vi "subFindAndSetSourcePath.vi"(4 "Name":string, 6 "ProjectItem path":path, 7 "Owning project":path, 9 "Skip":bool, 11 "Project items in":T1) -> (1 "Found":bool, 2 "Item found":refnum<class "ProjectItem.lvclass">[](array[class]), 3 "Project items out":T1)   [LabVIEW 2020, in "SolutionBuilder.lvlib" / "SolutionBuilder.lvclass"]
uses:
  SolutionBuilder.lvclass
  ProjectItem/ProjectItem.lvclass
  ProjectItemMap.ctl
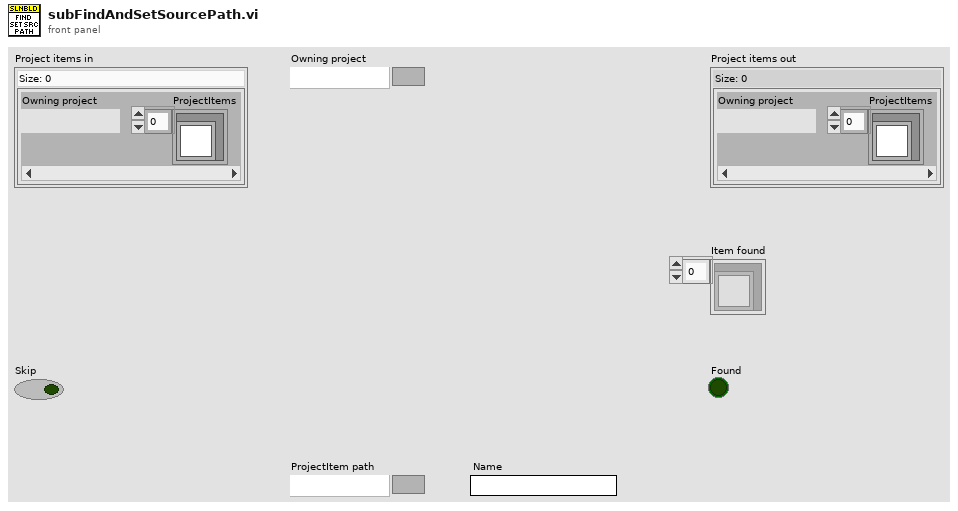
[diagram p1: front panel]
types:
  T1 = typedef "SolutionBuilder.lvlib/SolutionBuilder.lvclass/ProjectItemMap.ctl" = map{path, refnum<class "ProjectItem.lvclass">[]}
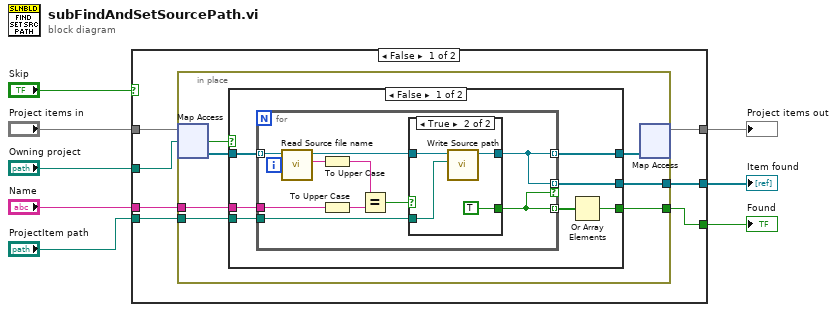
[diagram p0: block diagram]
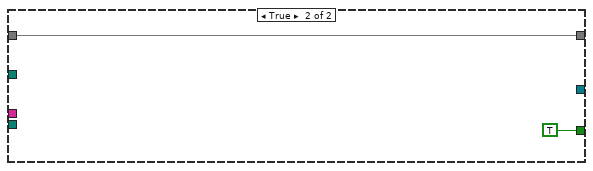
[diagram p4: hidden frame]
diagram:
  n1 = case shown="False" "Skip" {
    tunnel: "Project items in" -> [w15 w47]
    tunnel: "Name" -> [w14 _]
    tunnel: "ProjectItem path" -> [w13 _]
    tunnel: [w12 w47] -> w5
    tunnel: [w11 _] -> w7
    tunnel: [w10 TRUE] -> w8
    tunnel: "Owning project" -> [w9 _]
    frame False {
      n2 = in-place {
        in-place-border: w14 -> [w22]
        in-place-border: w13 -> [w21]
        in-place-border: [w17] -> w11
        in-place-border: [w16] -> w10
        n3 = in-place-map #1(w15, w9) -> (w19:refnum<class "ProjectItem.lvclass">[], w20:bool)  [unwired: 1 in]
        n4 = case shown="False" w20 {
          tunnel: w22 -> [w28 _]
          tunnel: w21 -> [w27 _]
          tunnel: w19 -> [w29 w45]
          tunnel: [w26 w45] -> w18
          tunnel: [w25 _] -> w17
          tunnel: [w23 _] -> w16
          frame False {
            n5 = for {
              tunnel: w29 -> [w39] mode=indexing
              tunnel: w28 -> [w35]
              tunnel: [w31] -> w26 mode=indexing
              tunnel: w27 -> [w32]
              tunnel: [w31] -> w25 mode=indexing if=w30
              tunnel: [w30] -> w24 mode=indexing
              n6 = call-dynamic "Read Source file name.vi"("ProjectItem in"=w39) -> ("Source file name"=w38:string, "ProjectItem out"=w34:refnum<class "ProjectItem.lvclass">)  [unwired: 9 in]
              n7 = To Upper Case(1:w38) -> (0:w37:string)
              n8 = To Upper Case(1:w35) -> (0:w36:string)
              n9 = Equal?(x=w37, y=w36) -> (x = y?=w33:bool)
              n10 = case shown="True" w33 {
                tunnel: w34 -> [w40 w44]
                tunnel: w32 -> [_ w43]
                tunnel: [w40 w42] -> w31
                tunnel: [_ TRUE] -> w30
                frame False {
                }
                frame True {
                  n11 = call-dynamic "Write Source path.vi"("Source path"=w43, "ProjectItem in"=w44) -> ("ProjectItem out"=w42:refnum<class "ProjectItem.lvclass">)  [unwired: 9 in]
                }
              }
            }
            n12 = Or Array Elements(Boolean array=w24) -> (logical OR=w23:bool)
          }
          frame True {
          }
        }
        n13 = in-place-map #1(w18) -> (w12:T1)  [unwired: 1 in, 2 out]
      }
    }
    frame True {
    }
  }
  "Found" <- w8
  "Item found" <- w7
  "Project items out" <- w5
